vi "notifier with timeout.vi"(6 "notify close?":refnum<vi>, 8 "Monitor":string, 9 "Timeout (ms)":i32=5000, 10 "Text Color":u32, 11 "String input":string) -> (0 "error out":errorcluster)   [LabVIEW 2015]
uses:
  <vilib>/Utility/miscctls.llb/LVPointTypeDef.ctl
panel:
  in  "Cancel Button":bool
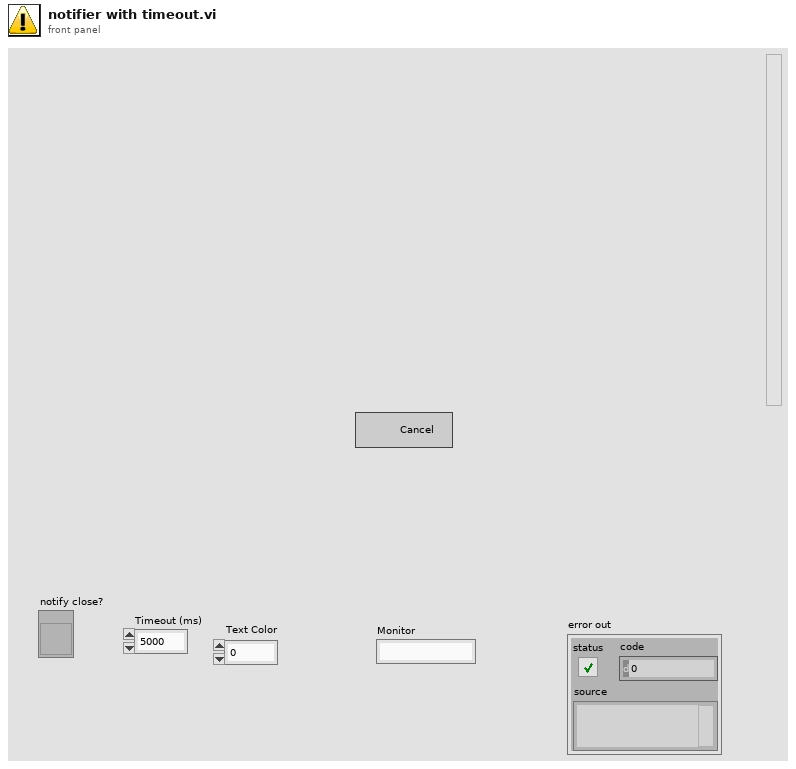
[diagram p1: front panel]
types:
  T1 = enum32{"Invalid", "Standard", "Closed", "Hidden", "Minimized", "Maximized"}
  T2 = typedef "LVPointTypeDef.ctl" = cluster{"Horizontal":i16, "Vertical":i16}
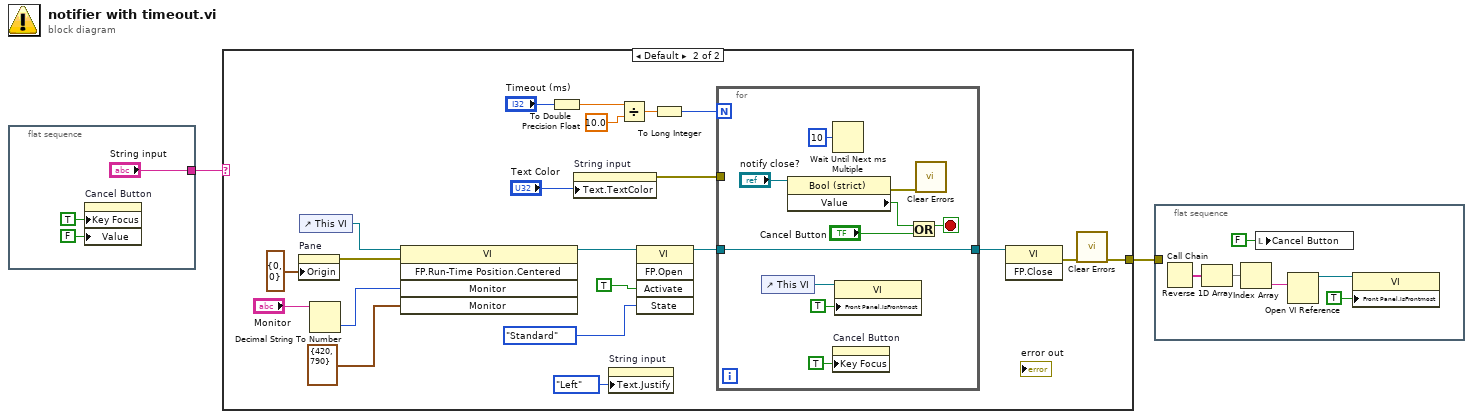
[diagram p0: block diagram]
diagram:
  n1 = flat-sequence {
    tunnel: ["String input"] -> w2
    frame #0 {
      n2 = property on="Cancel Button" class="Bool (strict)"("Key Focus"=TRUE, "Value"=FALSE ("Cancel Button")) -> ()  [unwired: 2 in, 2 out]
    }
  }
  n3 = case shown="Default" w2 {
    tunnel: [_ w6] -> w1
    frame "" {
    }
    frame Default {
      n4 = property on="Pane" class="Pane"("Origin"=T2 {"Horizontal"=0, "Vertical"=0}) -> (error out=w20:errorcluster)  [unwired: 2 in, 1 out]
      n5 = control-ref of="This VI"() -> (w23:refnum<vi>)
      n6 = Decimal String To Number(string="Monitor") -> (number=w21:i32)  [unwired: 2 in, 1 out]
      n7 = invoke class="VI" method="FP.Run-Time Position.Centered"(reference=w23, error in=w20, "Monitor"=w21, "Monitor"=cluster{"Height":i16, "Width":i16} {"Height"=420, "Width"=790} ("Size")) -> (reference out=w19:refnum<vi>)  [unwired: 1 in, 4 out]
      n8 = To Double Precision Float(number="Timeout (ms)") -> (double precision float=w10:dbl)
      n9 = property on="String input" class="Str"("Text.TextColor"="Text Color") -> (error out=w25:errorcluster)  [unwired: 2 in, 1 out]
      n10 = property on="String input" class="Str"("Text.Justify"=enum16{"Left", "Center", "Right"}."Left" ("Text.Justification")) -> ()  [unwired: 2 in, 2 out]
      n11 = Divide(x=w10, y=10.0) -> (x/y=w11:dbl)
      n12 = invoke class="VI" method="FP.Open"(reference=w19, "Activate"=TRUE ("Activate?"), "State"=T1."Standard") -> (reference out=w18:refnum<vi>)  [unwired: 2 in, 4 out]
      n13 = To Long Integer(number=w11) -> (32bit integer=w9:i32)
      n14 = for {
        N: w9 -> [_]
        tunnel: w25 -> [_]
        tunnel: w18 -> [w36]
        tunnel: [w36] -> w17
        stop <- w31 stop-if-true
        n15 = control-ref of="This VI"() -> (w29:refnum<vi>)
        n16 = property class="Bool (strict)"(reference="notify close?") -> (error out=w32:errorcluster, "Value"=w33:bool)  [unwired: 1 in, 1 out]
        n17 = Wait Until Next ms Multiple(millisecond multiple=u32 10) -> ()  [unwired: 1 out]
        n18 = property on="Cancel Button" class="Bool (strict)"("Key Focus"=TRUE) -> ()  [unwired: 2 in, 2 out]
        n19 = property class="VI"(reference=w29, "Front Panel.IsFrontmost"=TRUE ("Front Panel Window:Is Frontmost")) -> ()  [unwired: 1 in, 2 out]
        n20 = Or(x=w33, y="Cancel Button") -> (x .or. y?=w31:bool)
        n21 = call <vilib>:"Clear Errors.vi"("error in (no error)"=w32) -> ()  [unwired: 5 in, 2 out]
      }
      n22 = invoke class="VI" method="FP.Close"(reference=w17) -> (error out=w8:errorcluster)  [unwired: 2 in, 2 out]
      n23 = call <vilib>:"Clear Errors.vi"("error in (no error)"=w8) -> ("error out"=w6:errorcluster)  [unwired: 5 in, 1 out]
    }
  }
  n24 = flat-sequence {
    tunnel: w1 -> [_]
    frame #0 {
      n25 = Call Chain() -> (call chain=w41:string[])
      n26 = Reverse 1D Array(array=w41) -> (reversed array=w40:string[])
      n27 = Index Array(array=w40) -> (element=w42:string)  [unwired: 1 in]
      n28 = local write "Cancel Button"(FALSE ("Cancel Button")) -> ()
      n29 = Open VI Reference(vi path=w42) -> (vi reference=w39:refnum<vi>)  [unwired: 5 in, 1 out]
      n30 = property class="VI"(reference=w39, "Front Panel.IsFrontmost"=TRUE ("Front Panel Window:Is Frontmost")) -> ()  [unwired: 1 in, 2 out]
    }
  }
